vi "S30c_dll Close Com.vi"(4 "error in":errorcluster) -> (0 "error out":errorcluster)   [LabVIEW 2014, in "K_S30c_dll.lvlib"]
uses:
  K_S30c_dll.lvlib
  s30c.dll
panel:
  # "write ROM F35"
  # "Close ComPort\nusing s30c.dll. \nComPort is automatic closed, if you open an  other ComPort\nor if the dll is removed from the Memory. \nKeller AG für Druckmesstechnik\n29.5.08 b.v."
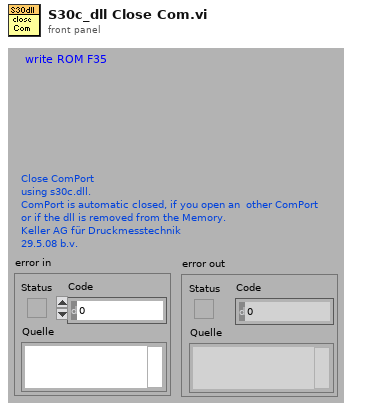
[diagram p1: front panel]
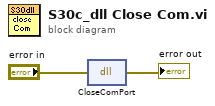
[diagram p0: block diagram]
diagram:
  n1 = dll-call lib="PTH2Labs EworkSINOPEC北控自动相渗software2.08.5_dlls30c.dll" fn="CloseComPort"(error in="error in") -> (error out=→"error out":errorcluster)  [unwired: 3 in, 1 out]
